vi "SVT Decimated Exp Avg Level (N Ch).vi"(6 "restart averaging (F)":bool, 7 "decimation factor":i32=-1, 8 "error in (no error)":errorcluster, 9 "time constant [ms]":dbl=125.0 format="%.2f", 10 "exponential mode":enum16{"Slow", "Fast", "Impulse", "Custom"}(ring)=enum."Fast", 11 "scaled signals [EU]":waveform(dbl)[](array[waveform])) -> (0 "error out":errorcluster, 1 "actual time constant [ms]":dbl=nan format="%.2f", 2 "unit labels":string[](array[string]), 3 "decimated exp avg levels [EU rms]":waveform(dbl)[](array[waveform]), 5 "actual decimation factor":i32=-1)   [LabVIEW 2017]
doc: "Computes the exponential average level of <B>scaled signal [EU]</B> or <B>even angle signal [EU]</B> and then decimates the level signal by <B>decimation factor</B>. You can use this polymorphic VI to compute the exponential average level for a single channel or for N channels or for a single channel or N channels of angular resampled data. The data type you wire to the <B>scaled signal [EU]</B> or <B>even angle signal [EU]</B> input determines the polymorphic instance to use."
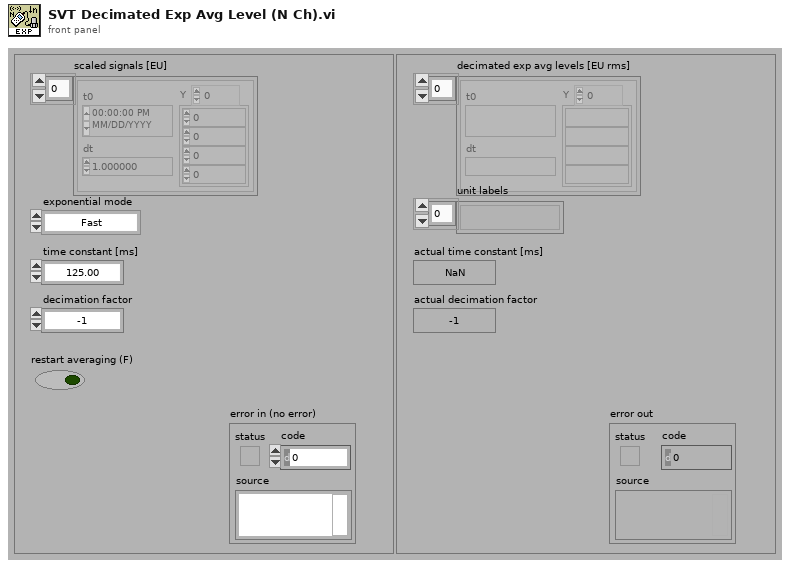
[diagram p1: front panel]
types:
  T1 = enum16{"RMS", "Running RMS", "Exp avg  ", "Dec exp avg ", "Peak", "Crest"}
  T2 = enum16{"Reset filter", "Restart averaging", "Continue processing"}
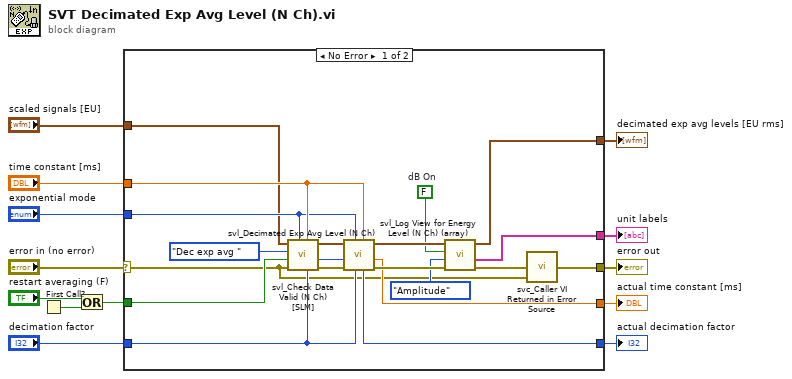
[diagram p0: block diagram]
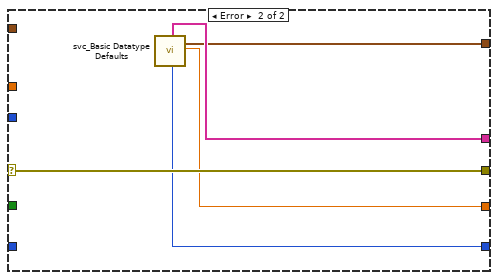
[diagram p2: hidden frame]
diagram:
  n1 = First Call?() -> (First Call?: T/F=w10:bool)
  n2 = Or(x="restart averaging (F)", y=w10) -> (x .or. y?=w9:bool)
  n3 = case shown="No Error" "error in (no error)" {
    selector: "error in (no error)" -> [w14 w38]
    tunnel: [w21 w38] -> w13
    tunnel: [w29 w37] -> w12
    tunnel: w9 -> [w19 _]
    tunnel: [w25 w36] -> w8
    tunnel: "time constant [ms]" -> [w24 _]
    tunnel: "decimation factor" -> [w20 _]
    tunnel: [w23 w35] -> w5
    tunnel: "exponential mode" -> [w22 _]
    tunnel: "scaled signals [EU]" -> [w17 _]
    tunnel: [w15 w34] -> w2
    frame No Error {
      w28 = FALSE  # dB On
      n4 = call <vilib>:"svl_Check Data Valid (N Ch) [SLM].vi"("decimation factor"=w20, "time constant [ms]"=w24, "exponential mode"=w22, "error in (no error)"=w14, "restart averaging (F)"=w19, "level analysis"=T1."Dec exp avg " ("Level Analysis"), "scaled signals [EU]"=w17) -> ("error out"=w33:errorcluster, "processing state"=w26:T2, "dup scaled signals [EU]"=w16:waveform(dbl)[])  [unwired: 2 in]
      n5 = call <vilib>:"svl_Decimated Exp Avg Level (N Ch).vi"("time constant"=w24, "decimation factor"=w20, "exponential mode"=w22, "error in (no error)"=w33, "processing state"=w26, "scaled signals"=w16) -> ("error out"=w32:errorcluster, "actual time constant [ms]"=w25:dbl, "scaled signals"=w31:waveform(dbl)[], "actual decimation factor"=w23:i32)  [unwired: 2 in]
      n6 = call <vilib>:"svl_Log View for Energy Level (N Ch) (array).vi"("error in (no error)"=w32, "view mode"=enum16{"Power", "Amplitude"}."Amplitude", "dB On (T)"=w28, "scaled signals"=w31) -> ("error out"=w30:errorcluster, "unit labels"=w29:string[], "scaled signals"=w15:waveform(dbl)[])  [unwired: 5 in]
      n7 = call <vilib>:"svc_Caller VI Returned in Error Source.vi"("warning input to caller"=w14, "error in (no error)"=w30) -> ("error out"=w21:errorcluster)  [unwired: 3 in]
    }
    frame Error {
      n8 = call <vilib>:"svc_Basic Datatype Defaults.vi"() -> ("empty array of strings"=w37:string[], "zero I32"=w35:i32, "empty array of waveforms"=w34:waveform(dbl)[], "NaN"=w36:dbl)  [unwired: 7 in, 9 out]
    }
  }
  "decimated exp avg levels [EU rms]" <- w2
  "actual time constant [ms]" <- w8
  "unit labels" <- w12
  "error out" <- w13
  "actual decimation factor" <- w5
